vi "quadratic equation solver using formula node.vi"() -> ()   [LabVIEW 2024]
panel:
  out "d":dbl
  out "root2":dbl
  out "root1":dbl
  in  "c":dbl
  in  "b":dbl
  in  "a":dbl
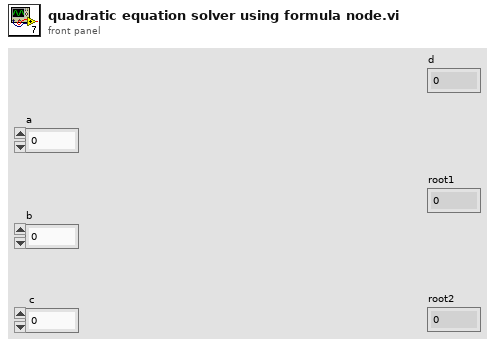
[diagram p1: front panel]
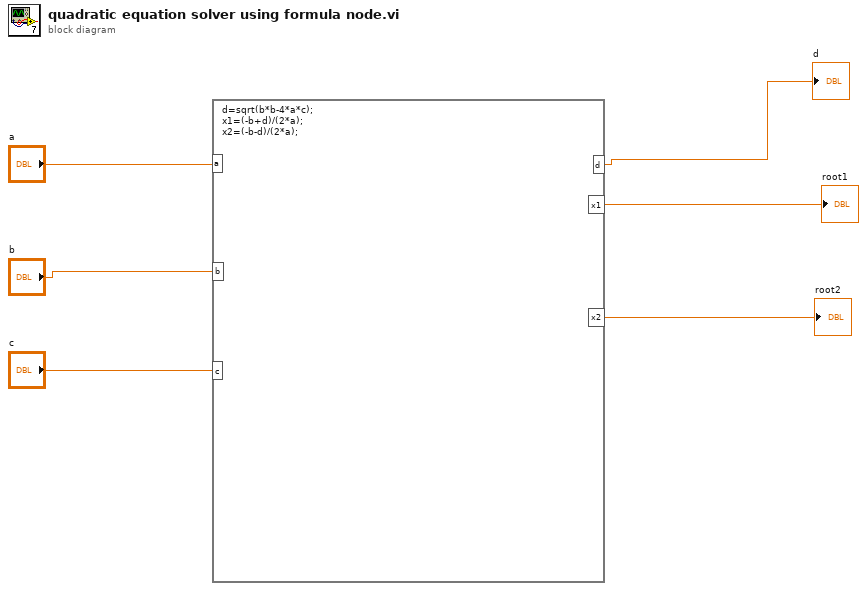
[diagram p0: block diagram]
diagram:
  n1 = formula code="d=sqrt(b*b-4*a*c);\nx1=(-b+d)/(2*a);\nx2=(-b-d)/(2*a);"("a"="a", "b"="b", "c"="c") -> ("x1"=→"root1":dbl, "x2"=→"root2":dbl, "d"=→"d":dbl)
